vi "TransformOperations.vi"() -> ()   [LabVIEW 2021]
panel:
  in  "Enum":T1(ring)
  in  "jd":dbl(slide) scale=1.0..10.0
  in  "id":dbl(slide) scale=0.0..10.0
  out "new picture":picture
  in  "Path":path
  # "Luis Eduardo Rodríguez Ramírez"
  # "Controles"
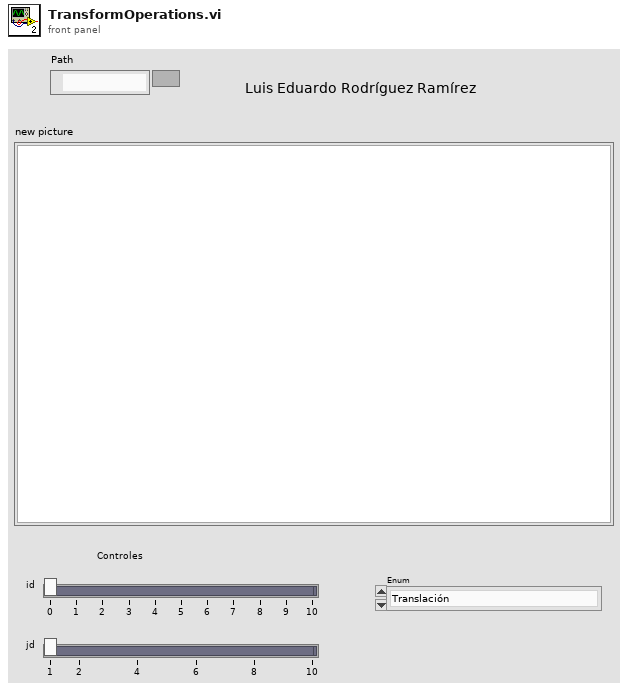
[diagram p1: front panel]
types:
  T1 = enum16{"Translación", "Rotación", "Escala", "Inclinación", "Perspectiva", "Deformaciones"}
  T2 = typedef "imagedata.ctl" = cluster{"image type":i32, "image depth":i32, "image":u8[], "mask":u8[], "colors":u32[], "Rectangle":cluster{"left":i16, "top":i16, "right":i16, "bottom":i16}}
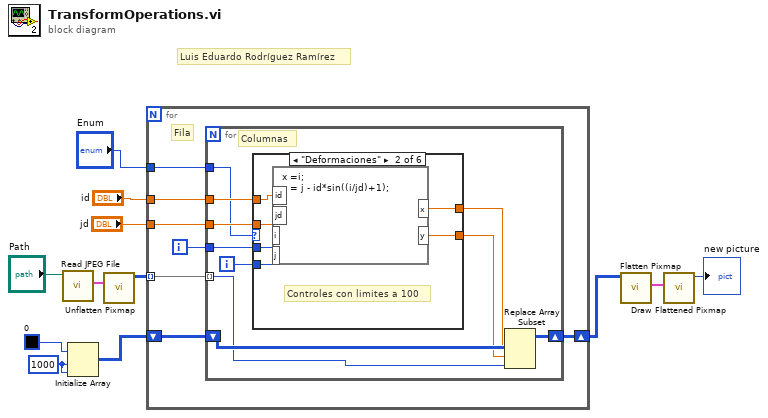
[diagram p0: block diagram]
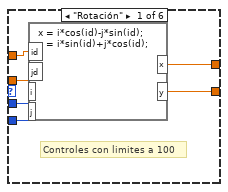
[diagram p2: hidden frame]
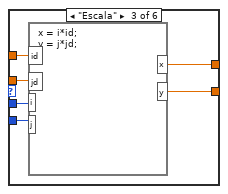
[diagram p3: hidden frame]
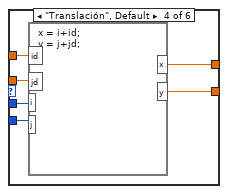
[diagram p4: hidden frame]
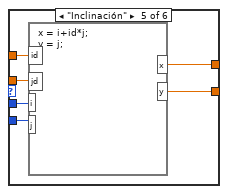
[diagram p5: hidden frame]
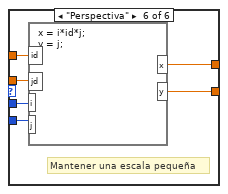
[diagram p6: hidden frame]
diagram:
  w7 = 1000 ("dimension size")
  # "Luis Eduardo Rodríguez Ramírez"
  n1 = call <vilib>:"Read JPEG File.vi"("path to JPEG file"="Path") -> ("image data"=w11:T2)  [unwired: 8 in, 2 out]
  n2 = Initialize Array(u32 0, w7, w7) -> (w5:u32[][])
  n3 = call <vilib>:"Unflatten Pixmap.vi"("image data"=w11) -> ("24-bit pixmap"=w8:u32[][])  [unwired: 4 in, 6 out]
  n4 = for {
    tunnel: w8 -> [w19] mode=indexing
    shift-right: [w17] -> w4
    shift-left: w5 -> [w18]
    tunnel: "id" -> [w16]
    tunnel: "jd" -> [w15]
    tunnel: "Enum" -> [w13]
    i -> [w14]
    # "Fila"
    n5 = for {
      tunnel: w19 -> [w21] mode=indexing
      shift-right: [w28] -> w17
      shift-left: w18 -> [w29]
      tunnel: w16 -> [w27]
      tunnel: w15 -> [w26]
      tunnel: w14 -> [w25]
      tunnel: w13 -> [w20]
      i -> [w24]
      # "Columnas"
      n6 = case shown="\"Deformaciones\"" w20 {
        tunnel: w27 -> [w35 w41 w47 w53 w59 w65]
        tunnel: w26 -> [w34 w40 w46 w52 w58 w64]
        tunnel: w25 -> [w33 w39 w45 w51 w57 w63]
        tunnel: w24 -> [w32 w38 w44 w50 w56 w62]
        tunnel: [w31 w37 w43 w49 w55 w61] -> w23
        tunnel: [w30 w36 w42 w48 w54 w60] -> w22
        frame "Rotación" {
          # "Controles con limites a 100"
          n7 = formula code="x = i*cos(id)-j*sin(id);\ny = i*sin(id)+j*cos(id);"("id"=w35, "jd"=w34, "i"=w33, "j"=w32) -> ("x"=w31:dbl, "y"=w30:dbl)
        }
        frame "Deformaciones" {
          # "Controles con limites a 100"
          n8 = formula code="x =i;\ny = j - id*sin((i/jd)+1);"("id"=w41, "jd"=w40, "i"=w39, "j"=w38) -> ("x"=w37:dbl, "y"=w36:dbl)
        }
        frame "Escala" {
          n9 = formula code="x = i*id;\ny = j*jd;"("id"=w47, "jd"=w46, "i"=w45, "j"=w44) -> ("x"=w43:dbl, "y"=w42:dbl)
        }
        frame "Translación", Default {
          n10 = formula code="x = i+id;\ny = j+jd;"("id"=w53, "jd"=w52, "i"=w51, "j"=w50) -> ("x"=w49:dbl, "y"=w48:dbl)
        }
        frame "Inclinación" {
          n11 = formula code="x = i+id*j;\ny = j;"("id"=w59, "jd"=w58, "i"=w57, "j"=w56) -> ("x"=w55:dbl, "y"=w54:dbl)
        }
        frame "Perspectiva" {
          # "Mantener una escala pequeña"
          n12 = formula code="x = i*id*j;\ny = j;"("id"=w65, "jd"=w64, "i"=w63, "j"=w62) -> ("x"=w61:dbl, "y"=w60:dbl)
        }
      }
      n13 = Replace Array Subset(array=w29, new element=w21, index (row)=w23, index (col)=w22) -> (w28:u32[][])
    }
  }
  n14 = call <vilib>:"Flatten Pixmap.vi"("24-bit pixmap"=w4) -> ("image data"=w10:T2)  [unwired: 10 in]
  n15 = call <vilib>:"Draw Flattened Pixmap.vi"("image data"=w10) -> ("new picture"=→"new picture":picture)  [unwired: 8 in]
